vi "Make Spacing Equal.vi"(1 "Points":T1[](array[typedef]), 2 "Smooth Points":dbl) -> (3 "Evenly spaced":T1[](array[typedef]))   [LabVIEW 2019, in "Tool Funnel.lvclass"]
uses:
  Tool Funnel.lvclass
  Tool Path/Tool Path.lvclass
  Parse/PathCommands/Point.ctl
  Parse/PathCommands/PathCommands.lvclass
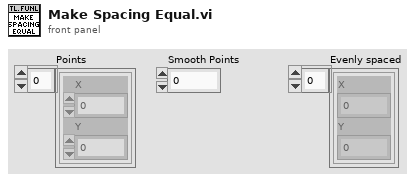
[diagram p1: front panel]
types:
  T1 = typedef "PathCommands.lvclass/Point.ctl" = cluster{"X":dbl, "Y":dbl}
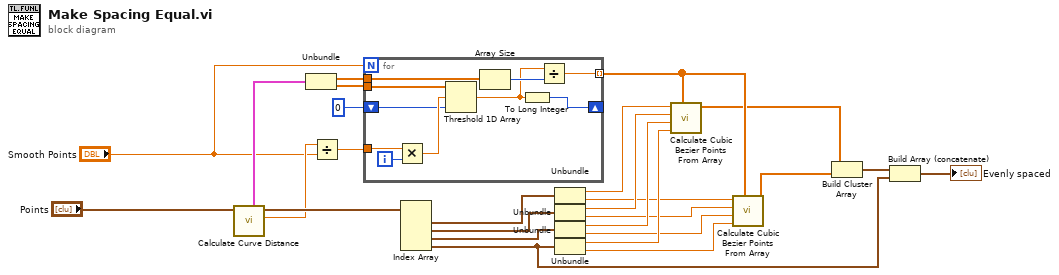
[diagram p0: block diagram]
diagram:
  n1 = call "Calculate Curve Distance.vi"("Points"="Points") -> ("Length"=w9:dbl, "Points Out"=w11:T1[], "Distance vs t"=w24:cluster{"t":dbl[], "Distance":dbl[]})  [unwired: 7 in, 1 out]
  n2 = Unbundle(w24) -> ("t"=w26:dbl[], "Distance"=w25:dbl[])
  n3 = Divide(x=w9, y="Smooth Points") -> (x/y=w10:dbl)
  n4 = for {
    N: "Smooth Points" -> [_]
    tunnel: w25 -> [w34]
    tunnel: w10 -> [w35]
    tunnel: w26 -> [w30]
    shift-right: [w32] -> _
    shift-left: 0 -> [w31]
    tunnel: [w27] -> w12 mode=indexing
    i -> [w36]
    n5 = Multiply(x=w35, y=w36) -> (x*y=w33:dbl)
    n6 = Threshold 1D Array(1:w31, 2:w33, 3:w34) -> (0:w28:dbl)
    n7 = Array Size(array=w30) -> (size(s)=w29:i32)
    n8 = To Long Integer(number=w28) -> (32bit integer=w32:i32)
    n9 = Divide(x=w28, y=w29) -> (x/y=w27:dbl)
  }
  n10 = Index Array(array=w11) -> (element #1=w21:T1, element #2=w22:T1, element #3=w23:T1, element #4=w1:T1)  [unwired: 4 in]
  n11 = Unbundle(w21) -> ("X"=w20:dbl, "Y"=w16:dbl)
  n12 = Unbundle(w22) -> ("X"=w19:dbl, "Y"=w15:dbl)
  n13 = Unbundle(w23) -> ("X"=w18:dbl, "Y"=w14:dbl)
  n14 = Unbundle(w1) -> ("X"=w17:dbl, "Y"=w13:dbl)
  n15 = call "Calculate Cubic Bezier Points From Array.vi"("t"=w12, "d"=w17, "c"=w18, "b"=w19, "a"=w20) -> ("f(t)"=w2:dbl[])  [unwired: 6 in]
  n16 = call "Calculate Cubic Bezier Points From Array.vi"("t"=w12, "d"=w13, "c"=w14, "b"=w15, "a"=w16) -> ("f(t)"=w3:dbl[])  [unwired: 6 in]
  n17 = Build Cluster Array(w2, w3) -> (w7:cluster{dbl, dbl}[])
  n18 = Build Array (concatenate)(w7, w1) -> (→"Evenly spaced":T1[])
